vi "Get UDP Info.vi"(5 "connection ID":refnum<k16>, 7 "Port Host":u16, 8 "error in":errorcluster, 9 "Port RT":u16, 10 "IP RT":string) -> (0 "error out":errorcluster)   [LabVIEW 2021, in "Main HMI.lvlib"]
doc: "_____\nCreated using DQMH Framework: Event Scripter 7.1.2.1547."
uses:
  Main HMI.lvlib
  Get UDP Info Argument--cluster.ctl
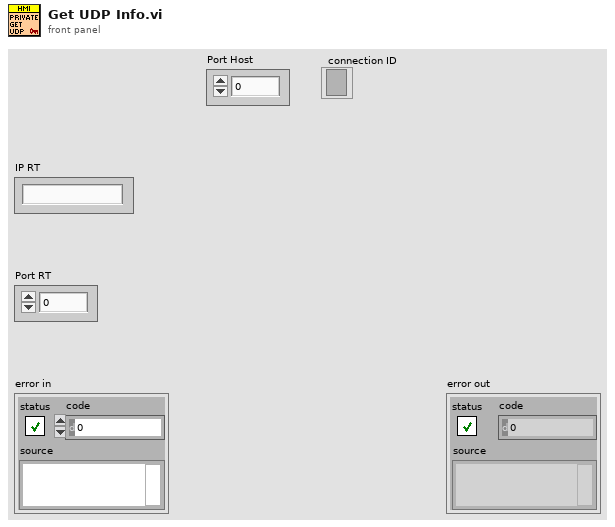
[diagram p1: front panel]
types:
  T1 = typedef "Main HMI.lvlib/Get UDP Info Argument--cluster.ctl" = cluster{"IP RT":string, "Port RT":u16, "Port Host":u16, "connection ID":refnum<k16>}
  T2 = typedef "Main HMI.lvlib/Request Events--cluster.ctl" = cluster{"Stop Module":refnum<user-event>, "Show Panel":refnum<user-event>, "Hide Panel":refnum<user-event>, "Get Module Execution Status":refnum<user-event>, "Show Diagram":refnum<user-event>, "Private.Open UDP Connection":refnum<user-event>, "Private.Get UDP Info":refnum<user-event>, "Private.Recording":refnum<user-event>}
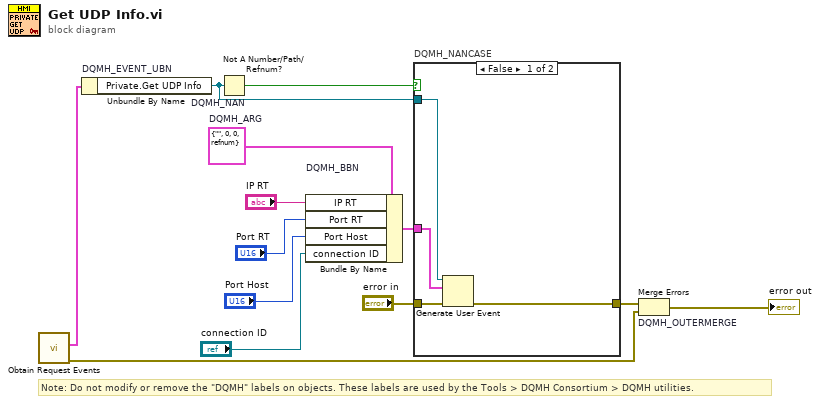
[diagram p0: block diagram]
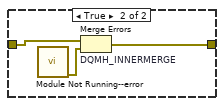
[diagram p2: hidden frame]
diagram:
  w7 = T1 {"IP RT"="", "Port RT"=0, "Port Host"=0, "connection ID"=refnum}  # DQMH_ARG
  # "Note: Do not modify or remove the \"DQMH\" labels on objects. These labels are used by the Tools > DQMH Consortium > DQMH utilities."
  n1 = call "Obtain Request Events.vi"() -> ("error out"=w2:errorcluster, "Main HMI Request Events"=w1:T2)  [unwired: 10 in]
  n2 = Unbundle By Name "DQMH_EVENT_UBN"(w1) -> ("Private.Get UDP Info"=w9:refnum<user-event>)
  n3 = Not A Number/Path/Refnum? "DQMH_NAN"(number/path/refnum=w9) -> (NaN/Path/Refnum?=w10:bool)
  n4 = Bundle By Name "DQMH_BBN"(cluster=w7, "IP RT"="IP RT", "Port RT"="Port RT", "Port Host"="Port Host", "connection ID"="connection ID") -> (w11:T1)
  n5 = case "DQMH_NANCASE" shown="False" w10 {
    tunnel: "error in" -> [w17 w20]
    tunnel: [w16 w19] -> w8
    tunnel: w9 -> [w15 _]
    tunnel: w11 -> [w14 _]
    frame False {
      n6 = Generate User Event(user event=w15, event data cluster=w14, error in=w17) -> (error out=w16:errorcluster)  [unwired: 1 in, 1 out]
    }
    frame True {
      n7 = call "Module Not Running--error.vi"() -> ("error out"=w18:errorcluster)  [unwired: 11 in]
      n8 = Merge Errors "DQMH_INNERMERGE"(w20, w18) -> (w19:errorcluster)
    }
  }
  n9 = Merge Errors "DQMH_OUTERMERGE"(w8, w2) -> (→"error out":errorcluster)
